vi "pointStringtoXY.vi"(11 "stringPoint":string) -> (2 "y":i32, 3 "x":i32)   [LabVIEW 2017]
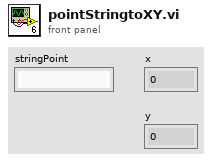
[diagram p1: front panel]
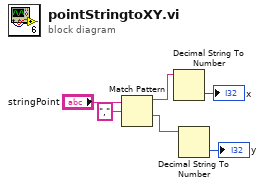
[diagram p0: block diagram]
diagram:
  n1 = Match Pattern(string="stringPoint", regular expression=",") -> (before substring=w4:string, after substring=w3:string)  [unwired: 1 in, 2 out]
  n2 = Decimal String To Number(string=w4) -> (number=→"x":i32)  [unwired: 2 in, 1 out]
  n3 = Decimal String To Number(string=w3) -> (number=→"y":i32)  [unwired: 2 in, 1 out]
